vi "Read File.vi"(8 "error in (no error)":errorcluster, 10 "Path in":path, 11 "Switch File Interface in":refnum<class "Switch File Interface.lvclass">) -> (0 "error out":errorcluster, 2 "SysDef":T1 {"Tree"."Properties"."Type" items=["K_STRING", "K_BOOL", "K_I32", "K_U32", "K_DOUBLE", "K_U64", "K_VARIANT", "K_DEPENDENTFILE", "K_DEPENDENTNODE", "K_DATASOURCENODE", "K_U16", "K_DBLARR", "K_U32ARR", "K_I32ARR", "K_STRINGARR", "K_DICTIONARY", "K_DICTIONARYARR"]})   [LabVIEW 2018, in "Switch System Explorer.lvlib" / "Switch File Interface.lvclass"]
uses:
  Switch Configuration.llb/Switch File Interface.lvclass
  Switch Configuration.llb/Switch CD Configuration.lvclass
  Switch Configuration.llb/PXI Card Config.lvclass
  Switch Configuration.llb/SLSC Card Config.lvclass
  C:/Users/jennifer.platt/Documents/Switch-Custom-Device - Copy/Built/Switch/Windows/Switch Configuration.llb/Switch Card Config.lvclass
  Switch Configuration.llb/Constants.vi
  Switch Configuration.llb/Switch Card Config.lvclass
  Switch Configuration.llb/Switch Shared.lvlib
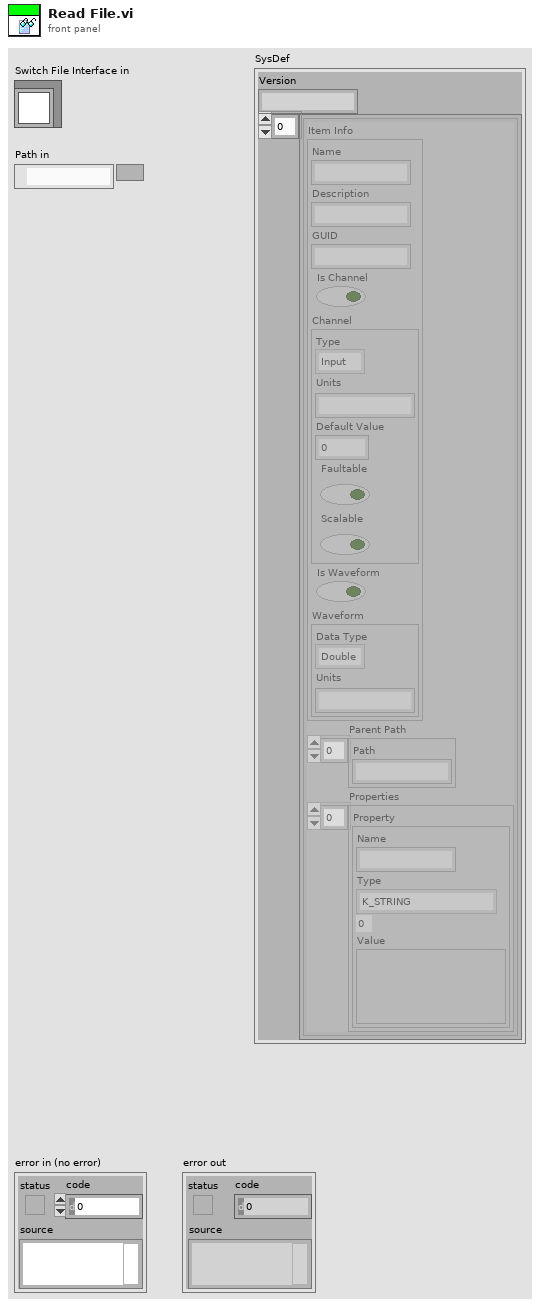
[diagram p1: front panel]
types:
  T1 = cluster{"Version":string, "Tree":cluster{"Item Info":cluster{"Name":string, "Description":string, "GUID":string, "Is Channel":bool, "Channel":cluster{"Type":enum16{"Input", "Output"}, "Units":string, "Default Value":dbl, "Faultable":bool, "Scalable":bool}, "Is Waveform":bool, "Waveform":cluster{"Data Type":enum16{"Double", "Complex Double"}, "Units":string}}, "Parent Path":string[], "Properties":cluster{"Name":string, "Type":i32, "Value":variant}[]}[]}
  T2 = cluster{"Startup and Shutdown Options":cluster{"Set all values to default on startup":bool, "Stop execution on error":bool, "Set all values to default on exit":bool}, "Value out of range handling:":enum32{"default state", "maintain state", "Shutdown"}}
  T3 = cluster{"Name":string, "Type":i32, "Value":variant}
  T4 = cluster{"Name":string, "Type":i32, "Value":variant}[]
  T5 = cluster{"Name":string, "Description":string, "GUID":string, "Is Channel":bool, "Channel":cluster{"Type":enum16{"Input", "Output"}, "Units":string, "Default Value":dbl, "Faultable":bool, "Scalable":bool}, "Is Waveform":bool, "Waveform":cluster{"Data Type":enum16{"Double", "Complex Double"}, "Units":string}}
  T6 = cluster{"Item Info":cluster{"Name":string, "Description":string, "GUID":string, "Is Channel":bool, "Channel":cluster{"Type":enum16{"Input", "Output"}, "Units":string, "Default Value":dbl, "Faultable":bool, "Scalable":bool}, "Is Waveform":bool, "Waveform":cluster{"Data Type":enum16{"Double", "Complex Double"}, "Units":string}}, "Parent Path":string[], "Properties":cluster{"Name":string, "Type":i32, "Value":variant}[]}
  T7 = cluster{"Set all values to default on startup":bool, "Stop execution on error":bool, "Set all values to default on exit":bool}
  T8 = enum32{"default state", "maintain state", "Shutdown"}
  T9 = cluster{"Channel Group Name":string, "Channel Configs":cluster{"Channel Name":string, "State Configs":cluster{"State Value":dbl, "State Name":string, "Command Configs":cluster{"Card Alias":string, "Ch0/Relay":string, "Ch1":string, "Disconnect(F)/Connect(T)":bool}[]}[]}[]}[]
  T10 = cluster{"Type":enum16{"Input", "Output"}, "Units":string, "Default Value":dbl, "Faultable":bool, "Scalable":bool}
  T11 = cluster{"Channel Name":string, "State Configs":cluster{"State Value":dbl, "State Name":string, "Command Configs":cluster{"Card Alias":string, "Ch0/Relay":string, "Ch1":string, "Disconnect(F)/Connect(T)":bool}[]}[]}
  T12 = cluster{"Channel Name":string, "State Configs":cluster{"State Value":dbl, "State Name":string, "Command Configs":cluster{"Card Alias":string, "Ch0/Relay":string, "Ch1":string, "Disconnect(F)/Connect(T)":bool}[]}[]}[]
  T13 = cluster{"State Value":dbl, "State Name":string, "Command Configs":cluster{"Card Alias":string, "Ch0/Relay":string, "Ch1":string, "Disconnect(F)/Connect(T)":bool}[]}[]
  T14 = cluster{"State Value":dbl, "State Name":string, "Command Configs":cluster{"Card Alias":string, "Ch0/Relay":string, "Ch1":string, "Disconnect(F)/Connect(T)":bool}[]}
  T15 = cluster{"Local(F)/Remote(T)":bool, "Host IP":string, "Port":i32}
  T16 = cluster{"Device/Resource Name":string, "Alias":string, "Topology Name":string, "Driver Type":enum16{"PXI", "SLSC"}, "Route(F)/Relay(T)":bool, "Channel List":string[], "Relay List":string[], "Simulate?":bool, "SLSC Driver Settings":cluster{"Local(F)/Remote(T)":bool, "Host IP":string, "Port":i32}, "Continuous Reservation?":bool}
  T17 = cluster{"Item Info":cluster{"Name":string, "Description":string, "GUID":string, "Is Channel":bool, "Channel":cluster{"Type":enum16{"Input", "Output"}, "Units":string, "Default Value":dbl, "Faultable":bool, "Scalable":bool}, "Is Waveform":bool, "Waveform":cluster{"Data Type":enum16{"Double", "Complex Double"}, "Units":string}}, "Parent Path":string[], "Properties":cluster{"Name":string, "Type":i32, "Value":variant}[]}[]
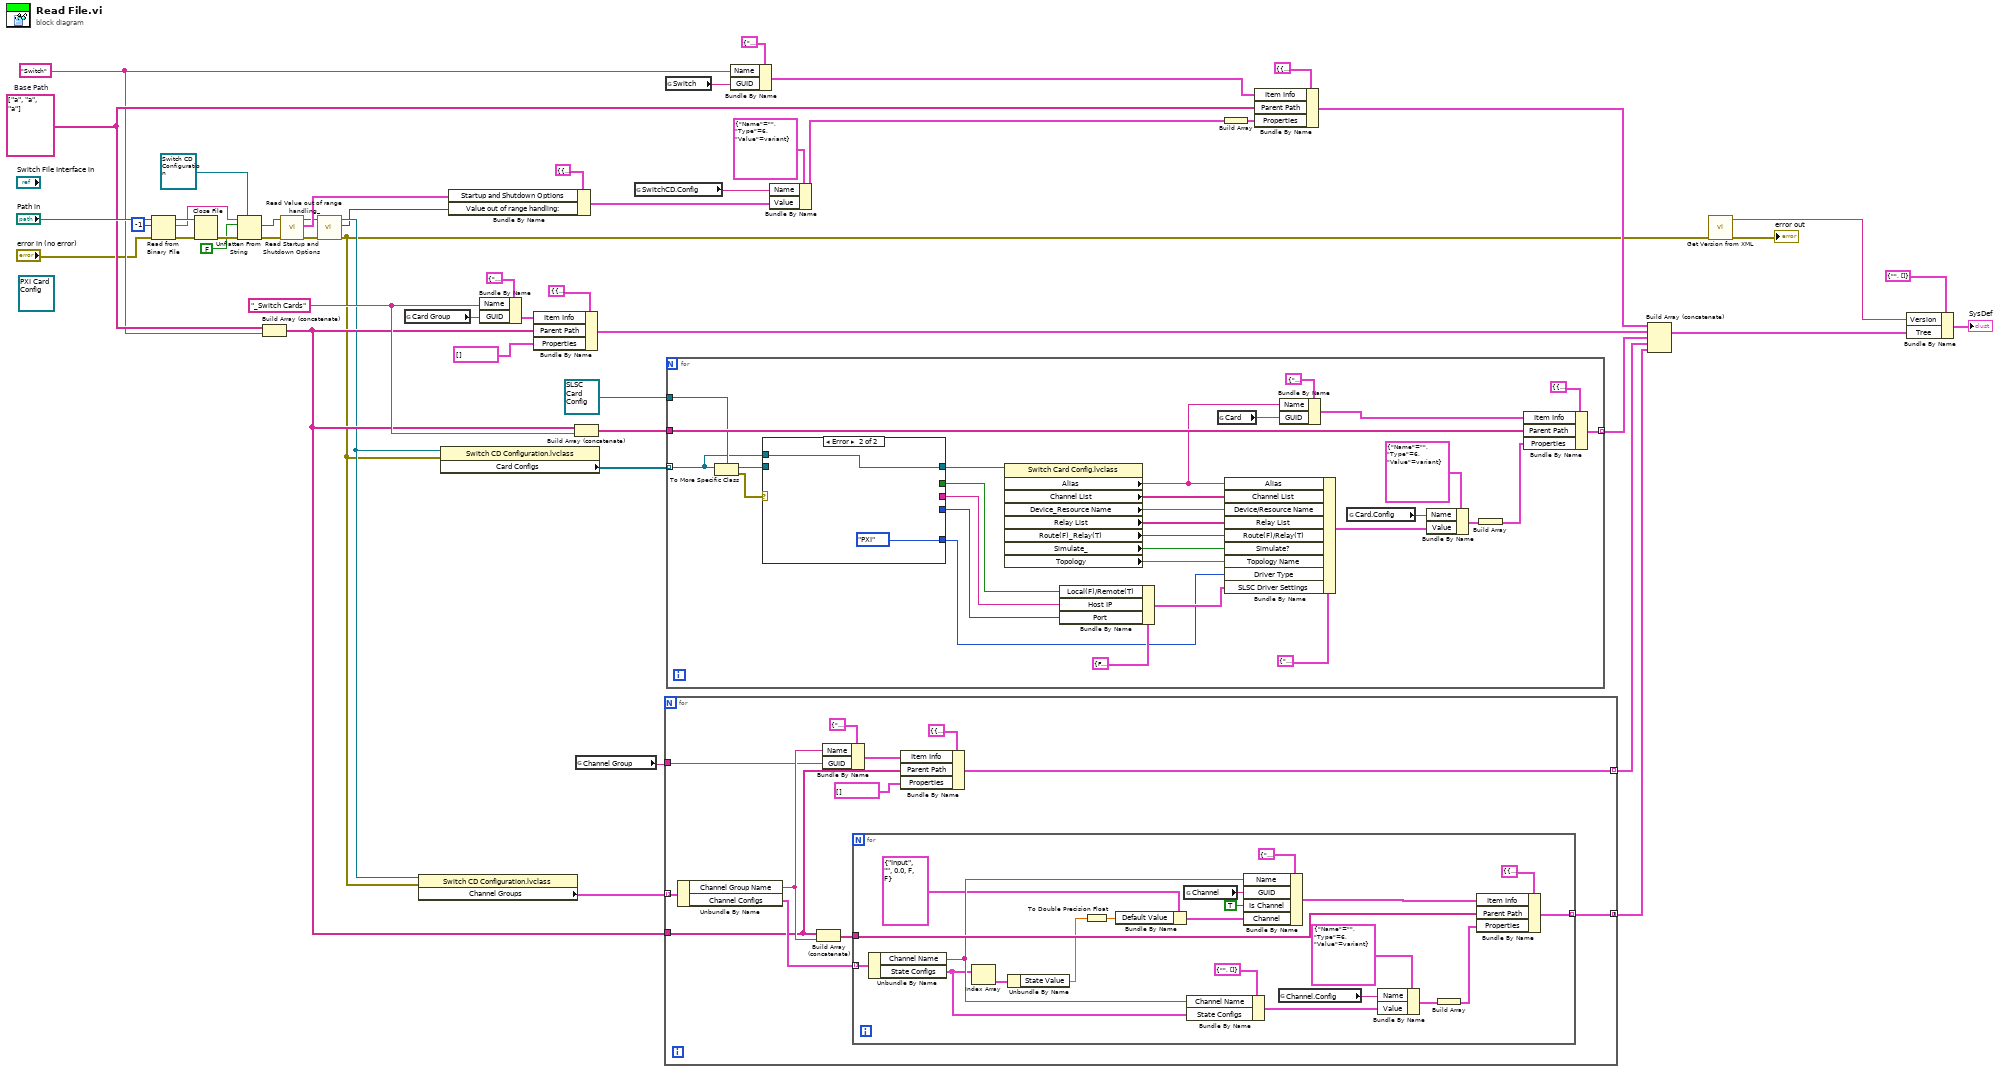
[diagram p0: block diagram]
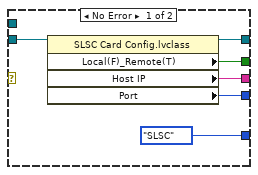
[diagram p2: hidden frame]
diagram:
  (unwired) refnum<class "PXI Card Config.lvclass"> refnum ("PXI Card Config.lvclass")
  w30 = "_Switch Cards" ("Name")
  w32 = "Switch" ("Name")
  w33 = string[] ["a", "a", "a"]  # Base Path
  n1 = Read from Binary File(8:"error in (no error)", 10:-1 ("count"), 11:"Path in") -> (0:w49:errorcluster, 2:w46:string, 3:w48:refnum<file>)  [unwired: 3 in, 1 out]
  n2 = Close File(refnum=w48, error in=w49) -> (error out=w47:errorcluster)  [unwired: 1 out]
  n3 = Unflatten From String(type=refnum<class "Switch CD Configuration.lvclass"> refnum ("Switch CD Configuration.lvclass"), binary string=w46, data includes array or string size? (T)=FALSE, error in (no error)=w47) -> (value=w9:refnum<class "Switch CD Configuration.lvclass">, error out=w8:errorcluster)  [unwired: 1 in, 1 out]
  n4 = Build Array (concatenate)(w33, w32) -> (w22:string[])
  n5 = call-dynamic "Read Startup and Shutdown Options.vi"("error in (no error)"=w8, "Switch CD Configuration in"=w9) -> ("error out"=w6:errorcluster, "Startup and Shutdown Options"=w10:T7, "Switch CD Configuration out"=w7:refnum<class "Switch CD Configuration.lvclass">)  [unwired: 7 in]
  n6 = call-dynamic "Read Value out of range handling_.vi"("error in (no error)"=w6, "Switch CD Configuration in"=w7) -> ("error out"=w2:errorcluster, "Value out of range handling:"=w12:T8, "Switch CD Configuration out"=w14:refnum<class "Switch CD Configuration.lvclass">)  [unwired: 7 in]
  n7 = global read "Constants.vi" "Card Group"() -> (w37:string)
  n8 = property class="Switch CD Configuration.lvclass"(reference=w14, error in=w2) -> ("Channel Groups"=w24:T9)  [unwired: 2 out]
  n9 = property class="Switch CD Configuration.lvclass"(reference=w14, error in=w2) -> ("Card Configs"=w31:refnum<class "Switch Card Config.lvclass">[])  [unwired: 2 out]
  n10 = Bundle By Name(cluster=T2 {"Startup and Shutdown Options"={"Set all values to default on startup"=FALSE, "Stop execution on error"=FALSE, "Set all values to default on exit"=FALSE}, "Value out of range handling:"=enum."default state"} ("Switch Device Data"), "Startup and Shutdown Options"=w10, "Value out of range handling:"=w12) -> (w11:T2)
  n11 = Bundle By Name(cluster=T5 {"Name"="", "Description"="", "GUID"="", "Is Channel"=FALSE, "Channel"={"Type"=enum."Input", "Units"="", "Default Value"=0.0, "Faultable"=FALSE, "Scalable"=FALSE}, "Is Waveform"=FALSE, "Waveform"={"Data Type"=enum."Double", "Units"=""}} ("Item Info"), "Name"=w30, "GUID"=w37) -> (w38:T5)
  n12 = Bundle By Name(cluster=T6 {"Item Info"={"Name"="", "Description"="", "GUID"="", "Is Channel"=FALSE, "Channel"={"Type"=enum."Input", "Units"="", "Default Value"=0.0, "Faultable"=FALSE, "Scalable"=FALSE}, "Is Waveform"=FALSE, "Waveform"={"Data Type"=enum."Double", "Units"=""}}, "Parent Path"=[], "Properties"=[]} ("TreeItem"), "Item Info"=w38, "Parent Path"=w22, "Properties"=T4 []) -> (w28:T6)
  n13 = Build Array (concatenate)(w22, w30) -> (w29:string[])
  n14 = global read "Constants.vi" "Channel Group"() -> (w20:string)
  n15 = global read "Constants.vi" "SwitchCD.Config"() -> (w15:string)
  n16 = for {
    tunnel: w24 -> [w63] mode=indexing
    tunnel: [w61] -> w23 mode=concatenating
    tunnel: w22 -> [w55]
    tunnel: [w53] -> w21 mode=indexing
    tunnel: w20 -> [w52]
    n17 = Unbundle By Name(w63) -> ("Channel Group Name"=w57:string, "Channel Configs"=w62:T12)
    n18 = Build Array (concatenate)(w55, w57) -> (w54:string[])
    n19 = Bundle By Name(cluster=T5 {"Name"="", "Description"="", "GUID"="", "Is Channel"=FALSE, "Channel"={"Type"=enum."Input", "Units"="", "Default Value"=0.0, "Faultable"=FALSE, "Scalable"=FALSE}, "Is Waveform"=FALSE, "Waveform"={"Data Type"=enum."Double", "Units"=""}} ("Item Info"), "Name"=w57, "GUID"=w52) -> (w60:T5)
    n20 = for {
      tunnel: w62 -> [w72] mode=indexing
      tunnel: [w74] -> w61 mode=indexing
      tunnel: w54 -> [w73]
      n21 = Unbundle By Name(w72) -> ("Channel Name"=w71:string, "State Configs"=w66:T13)
      n22 = Index Array(array=w66) -> (element=w65:T14)  [unwired: 1 in]
      n23 = Unbundle By Name(w65) -> ("State Value"=w64:dbl)
      n24 = To Double Precision Float(number=w64) -> (double precision float=w67:dbl)
      n25 = Bundle By Name(cluster=T10 {"Type"=enum."Input", "Units"="", "Default Value"=0.0, "Faultable"=FALSE, "Scalable"=FALSE} ("Channel"), "Default Value"=w67) -> (w68:T10)
      n26 = global read "Constants.vi" "Channel"() -> (w82:string)
      n27 = Bundle By Name(cluster=T11 {"Channel Name"="", "State Configs"=[]} ("Channel Config"), "Channel Name"=w71, "State Configs"=w66) -> (w77:T11)
      n28 = Bundle By Name(cluster=T5 {"Name"="", "Description"="", "GUID"="", "Is Channel"=FALSE, "Channel"={"Type"=enum."Input", "Units"="", "Default Value"=0.0, "Faultable"=FALSE, "Scalable"=FALSE}, "Is Waveform"=FALSE, "Waveform"={"Data Type"=enum."Double", "Units"=""}} ("Item Info"), "Name"=w71, "GUID"=w82, "Is Channel"=TRUE, "Channel"=w68) -> (w83:T5)
      n29 = global read "Constants.vi" "Channel.Config"() -> (w78:string)
      n30 = Bundle By Name(cluster=T3 {"Name"="", "Type"=6, "Value"=variant} ("Property"), "Name"=w78, "Value"=w77) -> (w76:T3)
      n31 = Build Array(w76) -> (w75:T4)
      n32 = Bundle By Name(cluster=T6 {"Item Info"={"Name"="", "Description"="", "GUID"="", "Is Channel"=FALSE, "Channel"={"Type"=enum."Input", "Units"="", "Default Value"=0.0, "Faultable"=FALSE, "Scalable"=FALSE}, "Is Waveform"=FALSE, "Waveform"={"Data Type"=enum."Double", "Units"=""}}, "Parent Path"=[], "Properties"=[]} ("TreeItem"), "Item Info"=w83, "Parent Path"=w73, "Properties"=w75) -> (w74:T6)
    }
    n33 = Bundle By Name(cluster=T6 {"Item Info"={"Name"="", "Description"="", "GUID"="", "Is Channel"=FALSE, "Channel"={"Type"=enum."Input", "Units"="", "Default Value"=0.0, "Faultable"=FALSE, "Scalable"=FALSE}, "Is Waveform"=FALSE, "Waveform"={"Data Type"=enum."Double", "Units"=""}}, "Parent Path"=[], "Properties"=[]} ("TreeItem"), "Item Info"=w60, "Parent Path"=w55, "Properties"=T4 []) -> (w53:T6)
  }
  n34 = global read "Constants.vi" "Switch"() -> (w40:string)
  n35 = for {
    tunnel: w31 -> [w87] mode=indexing
    tunnel: w29 -> [w110]
    tunnel: [w103] -> w27 mode=indexing
    tunnel: refnum<class "SLSC Card Config.lvclass"> refnum ("SLSC Card Config.lvclass") -> [w90]
    n36 = To More Specific Class(target class=w90, reference=w87) -> (specific class reference=w88:refnum<class "SLSC Card Config.lvclass">, error out=w89:errorcluster)  [unwired: 1 in]
    n37 = case shown="Error" w89 {
      tunnel: [w120 _] -> w94
      tunnel: [w119 _] -> w93
      tunnel: [w118 _] -> w95
      tunnel: [w117 w121] -> w91
      tunnel: w88 -> [w116 _]
      tunnel: [enum16{"PXI", "SLSC"}."SLSC" ("Driver Type") enum16{"PXI", "SLSC"}."PXI" ("Driver Type")] -> w86
      tunnel: w87 -> [_ w121]
      frame No Error {
        n38 = property class="SLSC Card Config.lvclass"(reference=w116) -> (reference out=w117:refnum<class "SLSC Card Config.lvclass">, "Local(F)_Remote(T)"=w120:bool, "Host IP"=w119:string, "Port"=w118:i32)  [unwired: 1 in, 1 out]
      }
      frame Error {
      }
    }
    n39 = property class="Switch Card Config.lvclass"(reference=w91) -> ("Alias"=w102:string, "Channel List"=w101:string[], "Device_Resource Name"=w85:string, "Relay List"=w100:string[], "Route(F)_Relay(T)"=w99:bool, "Simulate_"=w98:bool, "Topology"=w97:string)  [unwired: 1 in, 2 out]
    n40 = Bundle By Name(cluster=T15 {"Local(F)/Remote(T)"=FALSE, "Host IP"="", "Port"=0} ("SLSC Driver Settings"), "Local(F)/Remote(T)"=w94, "Host IP"=w93, "Port"=w95) -> (w92:T15)
    n41 = global read "Constants.vi" "Card"() -> (w112:string)
    n42 = Bundle By Name(cluster=T16 {"Device/Resource Name"="", "Alias"="", "Topology Name"="", "Driver Type"=enum."PXI", "Route(F)/Relay(T)"=FALSE, "Channel List"=[], "Relay List"=[], "Simulate?"=FALSE, "SLSC Driver Settings"={"Local(F)/Remote(T)"=FALSE, "Host IP"="", "Port"=0}, "Continuous Reservation?"=FALSE} ("Device Information"), "Alias"=w102, "Channel List"=w101, "Device/Resource Name"=w85, "Relay List"=w100, "Route(F)/Relay(T)"=w99, "Simulate?"=w98, "Topology Name"=w97, "Driver Type"=w86, "SLSC Driver Settings"=w92) -> (w107:T16)
    n43 = Bundle By Name(cluster=T5 {"Name"="", "Description"="", "GUID"="", "Is Channel"=FALSE, "Channel"={"Type"=enum."Input", "Units"="", "Default Value"=0.0, "Faultable"=FALSE, "Scalable"=FALSE}, "Is Waveform"=FALSE, "Waveform"={"Data Type"=enum."Double", "Units"=""}} ("Item Info"), "Name"=w102, "GUID"=w112) -> (w111:T5)
    n44 = global read "Constants.vi" "Card.Config"() -> (w106:string)
    n45 = Bundle By Name(cluster=T3 {"Name"="", "Type"=6, "Value"=variant} ("Property"), "Name"=w106, "Value"=w107) -> (w105:T3)
    n46 = Build Array(w105) -> (w104:T4)
    n47 = Bundle By Name(cluster=T6 {"Item Info"={"Name"="", "Description"="", "GUID"="", "Is Channel"=FALSE, "Channel"={"Type"=enum."Input", "Units"="", "Default Value"=0.0, "Faultable"=FALSE, "Scalable"=FALSE}, "Is Waveform"=FALSE, "Waveform"={"Data Type"=enum."Double", "Units"=""}}, "Parent Path"=[], "Properties"=[]} ("TreeItem"), "Item Info"=w111, "Parent Path"=w110, "Properties"=w104) -> (w103:T6)
  }
  n48 = Bundle By Name(cluster=T5 {"Name"="", "Description"="", "GUID"="", "Is Channel"=FALSE, "Channel"={"Type"=enum."Input", "Units"="", "Default Value"=0.0, "Faultable"=FALSE, "Scalable"=FALSE}, "Is Waveform"=FALSE, "Waveform"={"Data Type"=enum."Double", "Units"=""}} ("Item Info"), "Name"=w32, "GUID"=w40) -> (w39:T5)
  n49 = Bundle By Name(cluster=T3 {"Name"="", "Type"=6, "Value"=variant} ("Property"), "Name"=w15, "Value"=w11) -> (w17:T3)
  n50 = Build Array(w17) -> (w16:T4)
  n51 = Bundle By Name(cluster=T6 {"Item Info"={"Name"="", "Description"="", "GUID"="", "Is Channel"=FALSE, "Channel"={"Type"=enum."Input", "Units"="", "Default Value"=0.0, "Faultable"=FALSE, "Scalable"=FALSE}, "Is Waveform"=FALSE, "Waveform"={"Data Type"=enum."Double", "Units"=""}}, "Parent Path"=[], "Properties"=[]} ("TreeItem"), "Item Info"=w39, "Parent Path"=w33, "Properties"=w16) -> (w25:T6)
  n52 = Build Array (concatenate)(w25, w28, w27, w21, w23) -> (w26:T17)
  n53 = call "Get Version from XML.vi"("error in (no error)"=w2) -> ("error out"=→"error out":errorcluster, "node text"=w3:string)  [unwired: 9 in]
  n54 = Bundle By Name(cluster=T1 {"Version"="", "Tree"=[]} ("SysDef"), "Version"=w3, "Tree"=w26) -> (→"SysDef":T1)
